vi "Main.vi"(0 "ON/OFF":bool, 1 "Slave Address":u8 max=127 step=1 format="%x", 2 "Data":u8[](array[numeric]) format="%x", 5 "Write":bool, 7 "Mode":T2, 9 "Addressing Mode":T1, 11 "Error in":errorcluster) -> (15 "Error out":errorcluster)   [LabVIEW 2020, in "I2C Module.lvlib"]
doc: "This is the main application of the I2C module library which is used to generate and acquire the data of the SDA and SCL lines which act as a bus"
uses:
  I2C Module.lvlib
  Typedefs/Modes of i2c.ctl
  Typedefs/Addressing modes.ctl
  Typedefs/Queue operations.ctl
  Typedefs/Data Cluster.ctl
  Typedefs/Cluster mode.ctl
  Typedefs/Cluster addressing.ctl
panel:
  out "Digital Waveform Graph":digitaldata(graph) caption="I2C DATA"
  in  "Voltage":dbl=1.8 min=1.8 max=5.0 step=0.1
  in  "Frequency":u32=10 min=10 max=100 step=1
  in  "Read":bool
  # "INTER-INTEGRATED-CIRCUIT MODULE"
  # "I2C a two wire interface for wired communication between devices where mostly single master and multiple slaves \nare connected for transmission and reception of data. Basically not more than 50 devices are connected as there \nwill be introduction of bus capacitance and further data loss."
  # "OFF"
  # "ON"
  # "KHz"
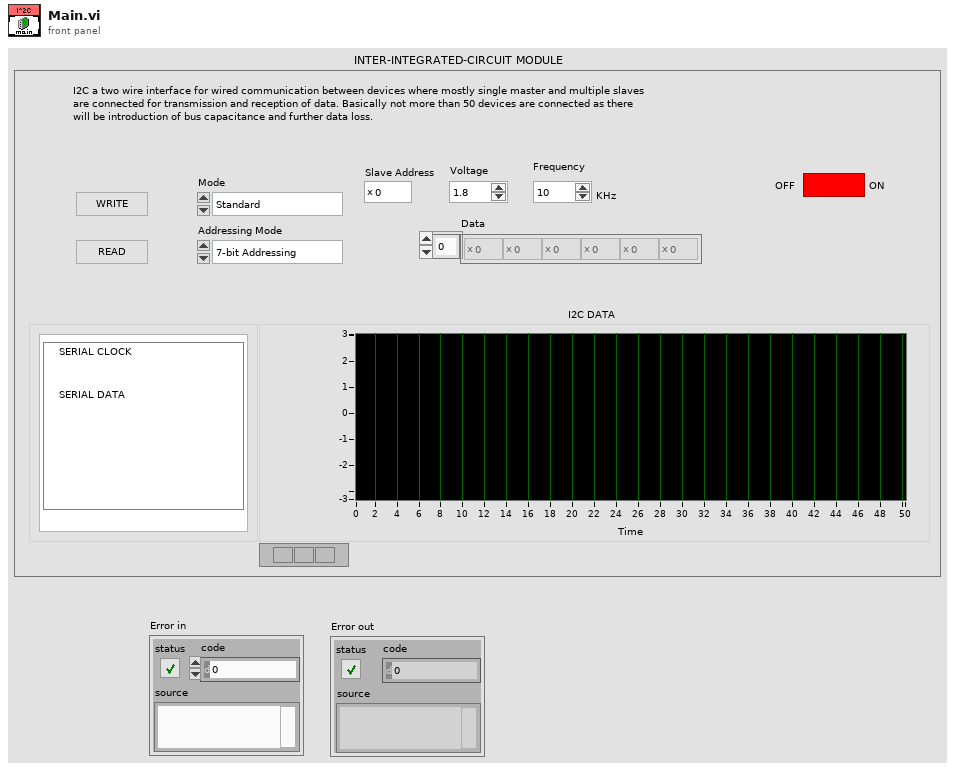
[diagram p1: front panel]
types:
  T1 = typedef "Addressing modes.ctl" = enum16{"7-bit Addressing", "10-bit Addressing"}
  T2 = typedef "Modes of i2c.ctl" = enum16{"Standard", "Fast Mode", "Fast Mode Plus"}
  T3 = typedef "Data Cluster.ctl" = cluster{"ON/OFF":bool, "Read":bool, "Stop":bool, "Ack":bool, "Nack":bool, "Mode":T4, "Addressing Mode":T5, "Frequency":u32, "Voltage":dbl, "SDA":bool[], "SCL":bool[], "Address":u8, "I2C DATA":dbl[], "I2C_DATA":dbl[][], "Enable":refnum<vi>[], "Disable":refnum<vi>[], "Write":bool, "I2C Digital":digitaldata, "Data":u8[], "Array update index":dbl}
  T4 = typedef "Cluster mode.ctl" = enum16{"Standard", "Fast Mode", "Fast Mode Plus"}
  T5 = typedef "Cluster addressing.ctl" = enum16{"7-bit Addressing", "10-bit Addressing"}
  T6 = typedef "I2C Module.lvlib/Queue operations.ctl" = enum16{"Create queue", " Enqueue N", "Enstack N", "Dequeue", "Flush", "Release"}
  T7 = enum8{"Enabled", "Disabled", "Disabled and Grayed Out"}
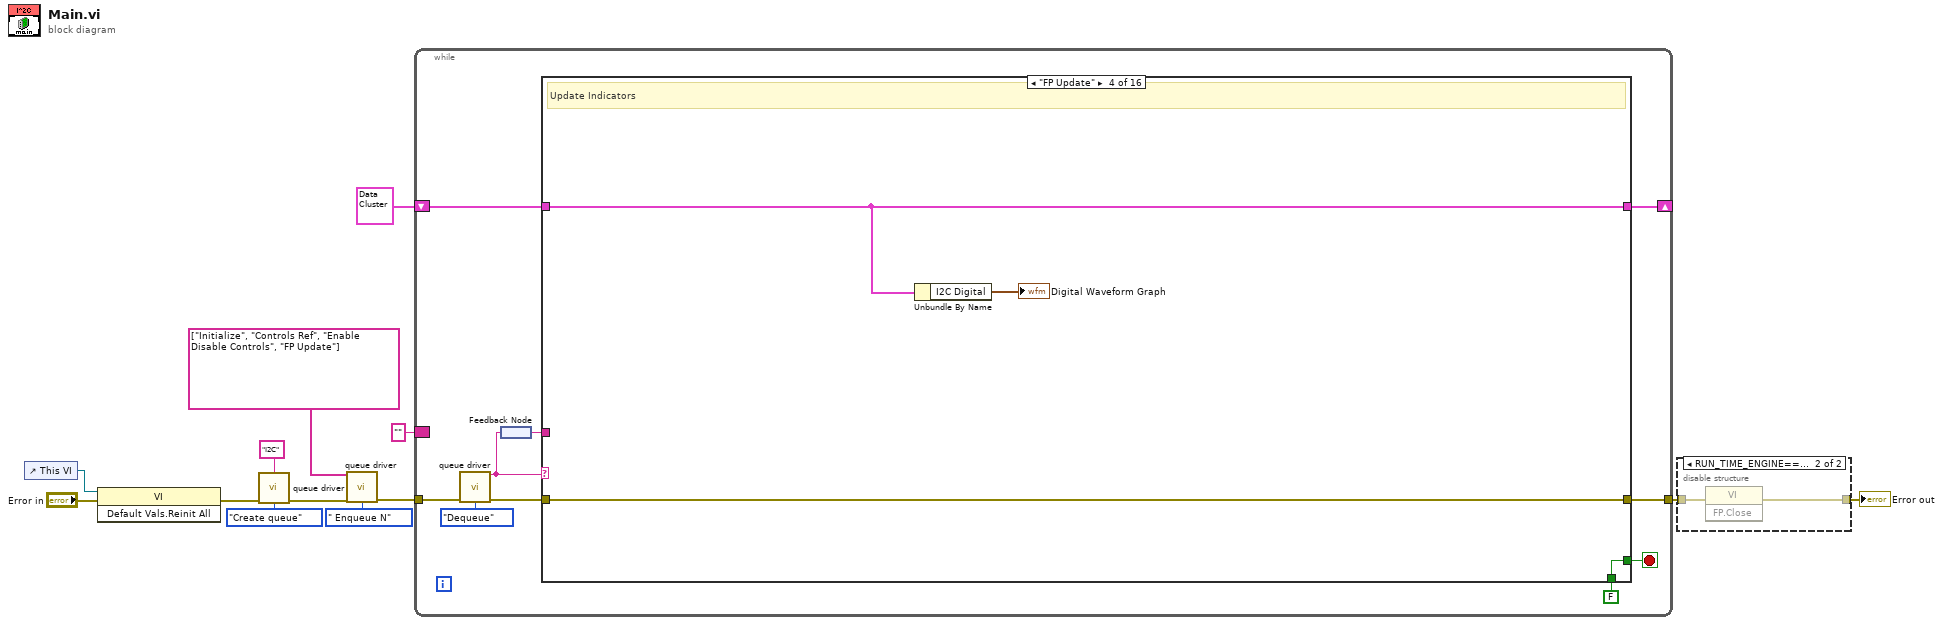
[diagram p0: block diagram]
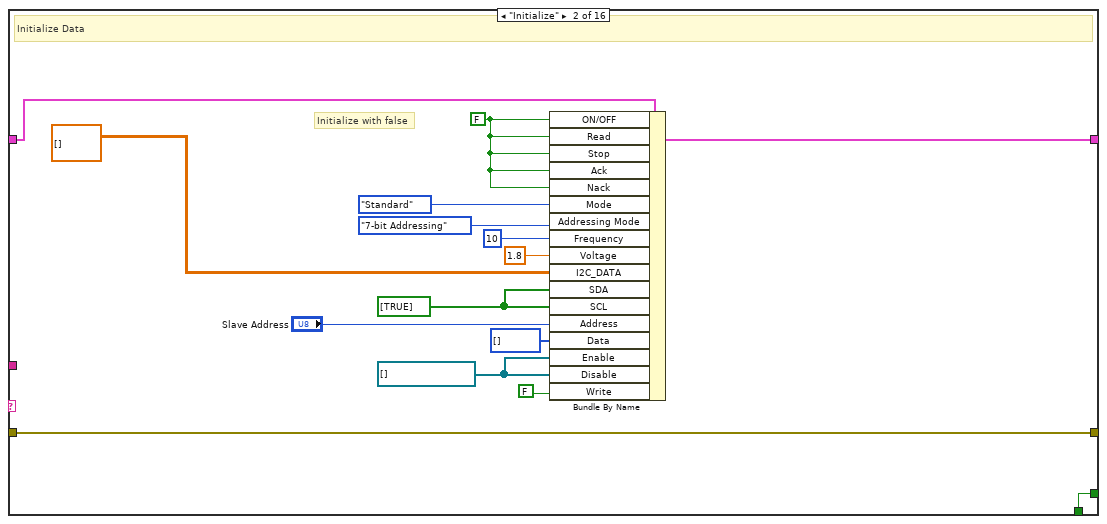
[diagram p4: hidden frame]
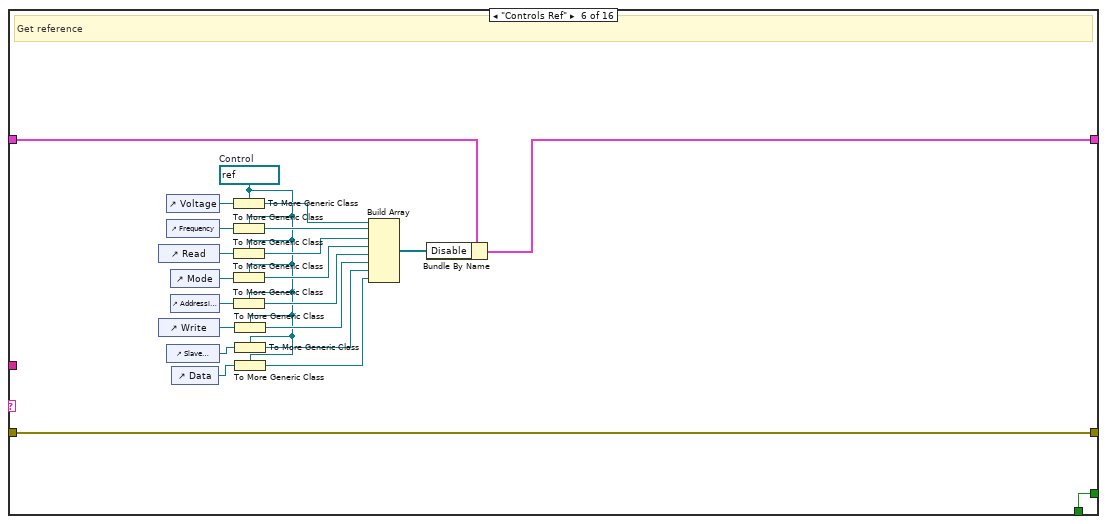
[diagram p7: hidden frame]
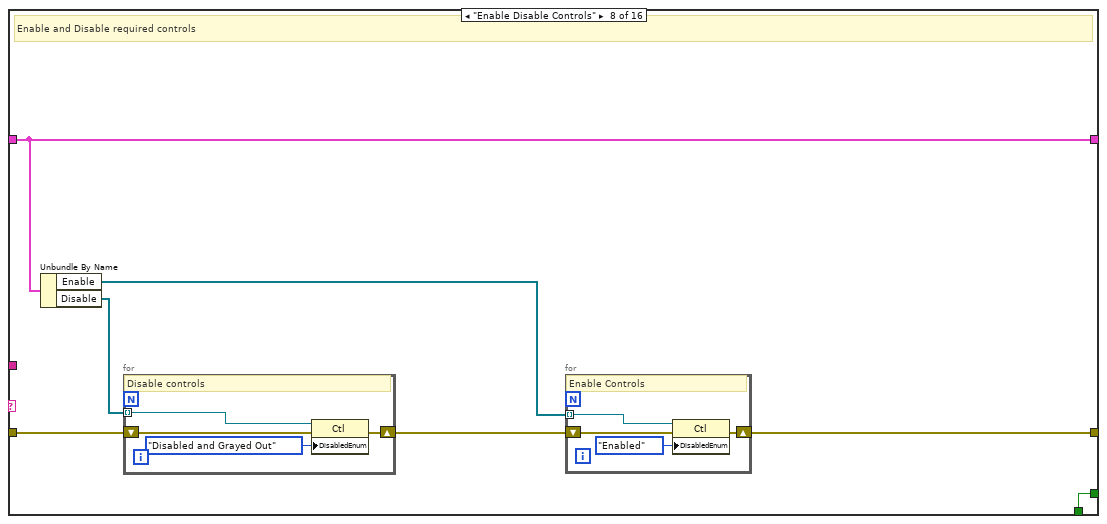
[diagram p9: hidden frame]
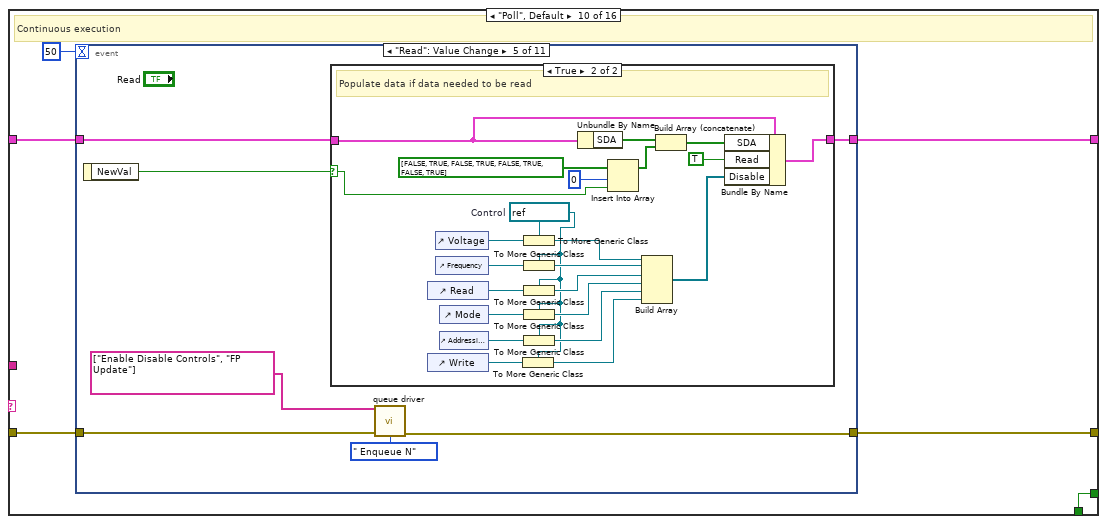
[diagram p11: hidden frame]
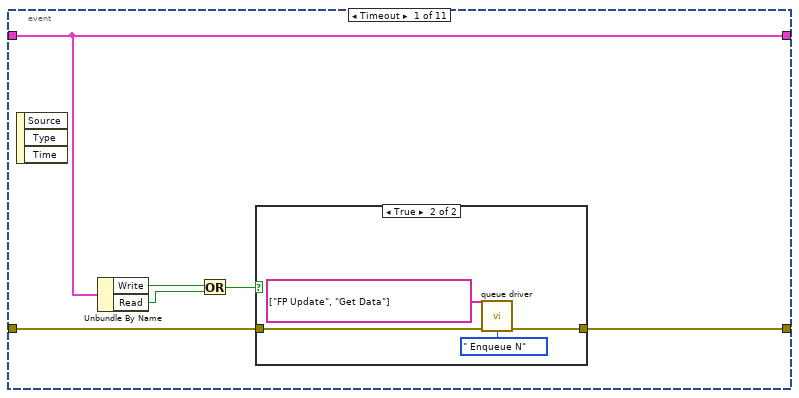
[diagram p12: hidden frame]
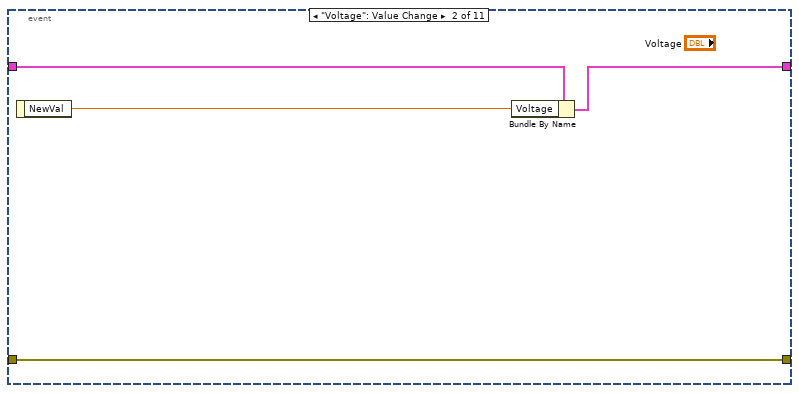
[diagram p14: hidden frame]
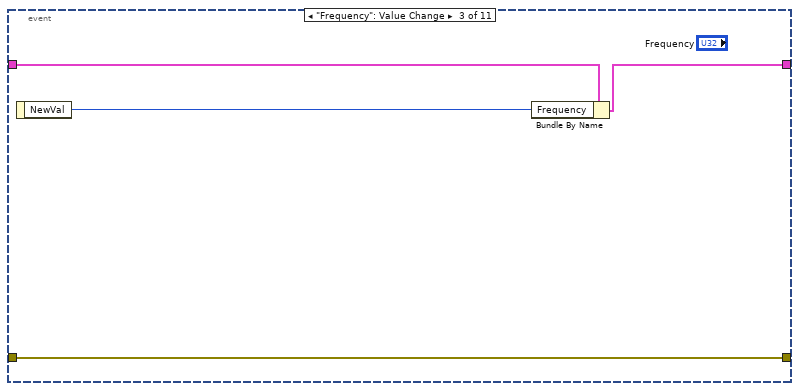
[diagram p15: hidden frame]
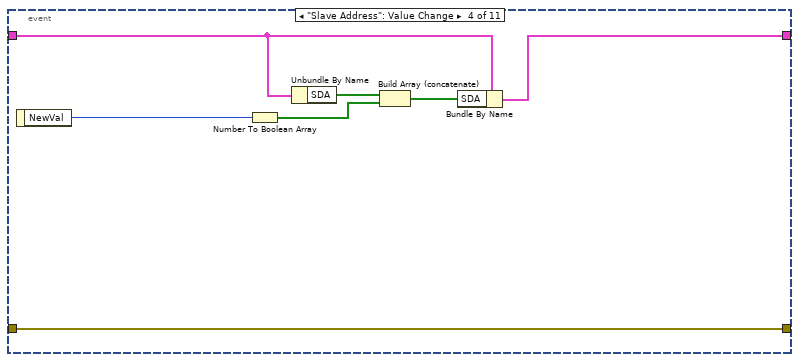
[diagram p16: hidden frame]
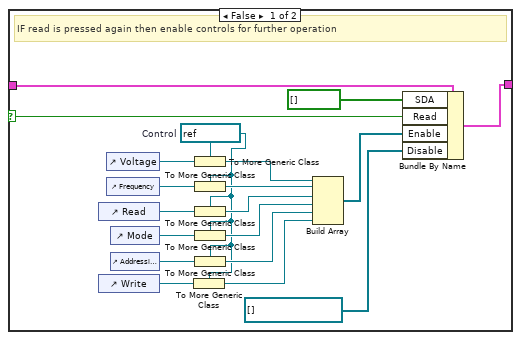
[diagram p17: hidden frame]
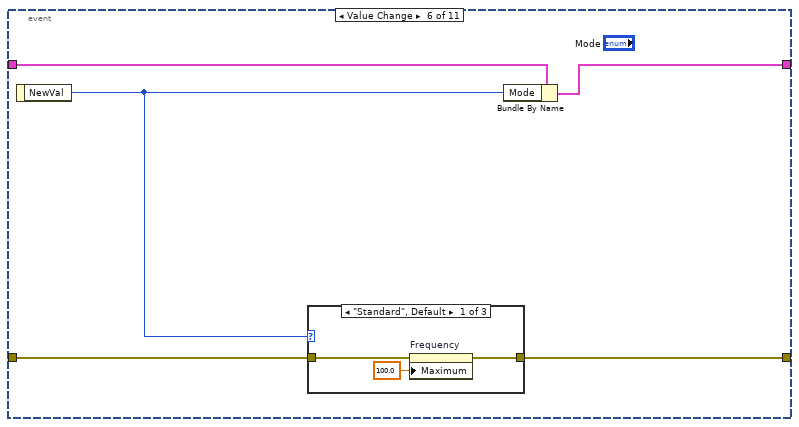
[diagram p18: hidden frame]
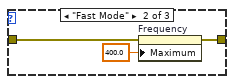
[diagram p19: hidden frame]
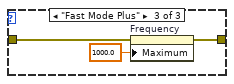
[diagram p20: hidden frame]
diagram:
  n1 = control-ref of="This VI"() -> (w12:refnum<vi>)
  n2 = invoke class="VI" method="Default Vals.Reinit All"(reference=w12, error in="Error in") -> (error out=w11:errorcluster)  [unwired: 1 in, 2 out]
  n3 = call "queue driver.vi"("Name"="I2C", "Error in"=w11, "Queue operations"=Queue_operations."Create queue") -> ("Error out"=w8:errorcluster)  [unwired: 11 in, 1 out]
  n4 = call "queue driver.vi"("Enqueue"=string[] ["Initialize", "Controls Ref", "Enable Disable Controls", "FP Update"], "Error in"=w8, "Queue operations"=Queue_operations." Enqueue N") -> ("Error out"=w6:errorcluster)  [unwired: 11 in, 1 out]
  n5 = while {
    tunnel: w6 -> [w22]
    border: "" ("Dequeued element") -> [_]
    tunnel: [w18] -> w2
    shift-right: [w15] -> _
    shift-left: T3 {"ON/OFF"=FALSE, "Read"=FALSE, "Stop"=FALSE, "Ack"=FALSE, "Nack"=FALSE, "Mode"=enum."Standard", "Addressing Mode"=enum."10-bit Addressing", "Frequency"=0, "Voltage"=0.0, "SDA"=[], "SCL"=[], "Address"=0, "I2C DATA"=[], "I2C_DATA"=[], "Enable"=[], "Disable"=[], "Write"=FALSE, "I2C Digital"={"transitions"=[], "data"=[]}, "Data"=[], "Array update index"=0.0} -> [w14]
    stop <- w17 stop-if-true
    n6 = call "queue driver.vi"("Error in"=w22, "Queue operations"=Queue_operations."Dequeue") -> ("Dequeued element"=w20:string, "Error out"=w19:errorcluster)  [unwired: 12 in]
    n7 = feedback-in #1(w20) -> ()
    n8 = feedback #1() -> (w21:string)
    n9 = case shown="\"FP Update\"" w20 {
      tunnel: w21 -> [_ _ _ _ _ _ _ _ _ _ _ _ _ w354 _ _]
      tunnel: w19 -> [w26 w41 w44 w48 w51 w73 w76 w81 w94 w98 w318 w341 w352 w356 w374 w379]
      tunnel: [w26 w41 w44 w48 w51 w73 w76 w80 w94 w99 w318 w341 w352 w355 w374 w377] -> w18
      tunnel: [w25 w40 w43 w47 w50 w72 w75 w83 w93 w97 w317 w340 w351 w366 w373 TRUE] -> w17
      tunnel: FALSE -> [w25 w40 w43 w47 w50 w72 w75 w83 w93 w97 w317 w340 w351 w366 w373 _]
      tunnel: [w24 w38 w42 w46 w49 w61 w74 w79 w92 w96 w316 w336 w350 w353 w372 w375] -> w15
      tunnel: w14 -> [w24 w39 w42 w46 w49 w62 w74 w79 w92 w95 w316 w337 w350 w353 w372 w375]
      frame "/***Initialize***/" {
      }
      frame "Initialize" {
        w28 = refnum<vi>[] [] ("Enable")
        w29 = bool[] [TRUE] ("SCL")
        w37 = FALSE ("ON/OFF")
        # "Initialize with false"
        # "Initialize Data"
        n10 = Bundle By Name(cluster=w39, "ON/OFF"=w37, "Read"=w37, "Stop"=w37, "Ack"=w37, "Nack"=w37, "Mode"=Cluster_mode."Standard", "Addressing Mode"=Cluster_addressing."7-bit Addressing", "Frequency"=u32 10, "Voltage"=1.8, "I2C_DATA"=dbl[][] [] ("x*y"), "SDA"=w29, "SCL"=w29, "Address"="Slave Address", "Data"=u8[] [], "Enable"=w28, "Disable"=w28, "Write"=FALSE ("Read/ Write")) -> (w38:T3)
      }
      frame "/***FP Related***/" {
      }
      frame "FP Update" {
        # "Update Indicators"
        n11 = Unbundle By Name(w46) -> ("I2C Digital"=→"Digital Waveform Graph":digitaldata)
      }
      frame "/***Controls ref***/" {
      }
      frame "Controls Ref" {
        w54 = refnum<vi> refnum  # Control
        # "Get reference"
        n12 = control-ref of="Read"() -> (w69:refnum<vi>)
        n13 = control-ref of="Write"() -> (w58:refnum<vi>)
        n14 = control-ref of="Voltage"() -> (w71:refnum<vi>)
        n15 = control-ref of="Frequency"() -> (w70:refnum<vi>)
        n16 = control-ref of="Slave Address"() -> (w56:refnum<vi>)
        n17 = control-ref of="Mode"() -> (w68:refnum<vi>)
        n18 = control-ref of="Addressing Mode"() -> (w67:refnum<vi>)
        n19 = control-ref of="Data"() -> (w55:refnum<vi>)
        n20 = To More Generic Class(target class=w54, reference=w71) -> (generic class reference=w66:refnum<vi>)
        n21 = To More Generic Class(target class=w54, reference=w70) -> (generic class reference=w65:refnum<vi>)
        n22 = To More Generic Class(target class=w54, reference=w69) -> (generic class reference=w64:refnum<vi>)
        n23 = To More Generic Class(target class=w54, reference=w68) -> (generic class reference=w63:refnum<vi>)
        n24 = To More Generic Class(target class=w54, reference=w67) -> (generic class reference=w59:refnum<vi>)
        n25 = To More Generic Class(target class=w54, reference=w58) -> (generic class reference=w57:refnum<vi>)
        n26 = To More Generic Class(target class=w54, reference=w56) -> (generic class reference=w53:refnum<vi>)
        n27 = To More Generic Class(target class=w54, reference=w55) -> (generic class reference=w52:refnum<vi>)
        n28 = Build Array(w66, w65, w64, w63, w59, w57, w53, w52) -> (w60:refnum<vi>[])
        n29 = Bundle By Name(cluster=w62, "Disable"=w60) -> (w61:T3)
      }
      frame "/***Enable Disable Controls***/" {
      }
      frame "Enable Disable Controls" {
        # "Enable and Disable required controls"
        n30 = Unbundle By Name(w79) -> ("Enable"=w78:refnum<vi>[], "Disable"=w77:refnum<vi>[])
        n31 = for {
          shift-right: [w90] -> w82
          shift-left: w81 -> [w91]
          tunnel: w77 -> [w88] mode=indexing
          # "Disable controls"
          n32 = property class="Ctl"(reference=w88, error in=w91, "DisabledEnum"=T7."Disabled and Grayed Out" ("Disabled")) -> (error out=w90:errorcluster)  [unwired: 1 out]
        }
        n33 = for {
          shift-right: [w86] -> w80
          shift-left: w82 -> [w87]
          tunnel: w78 -> [w84] mode=indexing
          # "Enable Controls"
          n34 = property class="Ctl"(reference=w84, error in=w87, "DisabledEnum"=T7."Enabled" ("Disabled")) -> (error out=w86:errorcluster)  [unwired: 1 out]
        }
      }
      frame "/***Application***/" {
      }
      frame "Poll", Default {
        # "Continuous execution"
        n35 = event shown="[4] \"Read\": Value Change" {
          selector: _ -> [_ _ _ _ _ _ _ _ _ _ _]
          dyn-events: _ -> [_ _ _ _ _ _ _ _ _ _ _]
          timeout: 50 -> [_ _ _ _ _ _ _ _ _ _ _]
          tunnel: [w105 w115 w119 w126 w128 w176 w193 w197 w241 w245 w311] -> w99
          tunnel: w98 -> [w106 w115 w119 w126 w129 w177 w193 w198 w241 w246 w312]
          tunnel: [w104 w113 w117 w123 w133 w179 w191 w200 w239 w242 w295] -> w96
          tunnel: w95 -> [w104 w114 w118 w124 w132 w180 w192 w194 w240 w243 w296]
          event Timeout {
            n36 = event-data() -> ()  [unwired: 1 in, 3 out]
            n37 = Unbundle By Name(w104) -> ("Write"=w103:bool, "Read"=w102:bool)
            n38 = Or(x=w103, y=w102) -> (x .or. y?=w101:bool)
            n39 = case shown="True" w101 {
              tunnel: w106 -> [w107 w110]
              tunnel: [w107 w109] -> w105
              frame False {
              }
              frame True {
                n40 = call "queue driver.vi"("Enqueue"=string[] ["FP Update", "Get Data"], "Error in"=w110, "Queue operations"=Queue_operations." Enqueue N") -> ("Error out"=w109:errorcluster)  [unwired: 11 in, 1 out]
              }
            }
          }
          event "Voltage": Value Change {
            n41 = event-data() -> ("NewVal"=w112:dbl)  [unwired: 1 in]
            n42 = Bundle By Name(cluster=w114, "Voltage"=w112) -> (w113:T3)
          }
          event "Frequency": Value Change {
            n43 = event-data() -> ("NewVal"=w116:u32)  [unwired: 1 in]
            n44 = Bundle By Name(cluster=w118, "Frequency"=w116) -> (w117:T3)
          }
          event "Slave Address": Value Change {
            n45 = event-data() -> ("NewVal"=w125:u8)  [unwired: 1 in]
            n46 = Number To Boolean Array(number=w125) -> (Boolean array=w120:bool[])
            n47 = Unbundle By Name(w124) -> ("SDA"=w122:bool[])
            n48 = Build Array (concatenate)(w122, w120) -> (w121:bool[])
            n49 = Bundle By Name(cluster=w124, "SDA"=w121) -> (w123:T3)
          }
          event "Read": Value Change {
            n50 = event-data() -> ("NewVal"=w131:bool)  [unwired: 1 in]
            n51 = case shown="True" w131 {
              selector: w131 -> [w150 w167]
              tunnel: [w151 w175] -> w133
              tunnel: w132 -> [w152 w168]
              frame False {
                w136 = refnum<vi> refnum  # Control
                # "IF read is pressed again then enable controls for further operation"
                n52 = control-ref of="Read"() -> (w139:refnum<vi>)
                n53 = control-ref of="Write"() -> (w147:refnum<vi>)
                n54 = control-ref of="Voltage"() -> (w141:refnum<vi>)
                n55 = control-ref of="Frequency"() -> (w140:refnum<vi>)
                n56 = control-ref of="Mode"() -> (w138:refnum<vi>)
                n57 = control-ref of="Addressing Mode"() -> (w137:refnum<vi>)
                n58 = To More Generic Class(target class=w136, reference=w147) -> (generic class reference=w148:refnum<vi>)
                n59 = To More Generic Class(target class=w136, reference=w141) -> (generic class reference=w146:refnum<vi>)
                n60 = To More Generic Class(target class=w136, reference=w140) -> (generic class reference=w145:refnum<vi>)
                n61 = To More Generic Class(target class=w136, reference=w139) -> (generic class reference=w144:refnum<vi>)
                n62 = To More Generic Class(target class=w136, reference=w138) -> (generic class reference=w143:refnum<vi>)
                n63 = To More Generic Class(target class=w136, reference=w137) -> (generic class reference=w142:refnum<vi>)
                n64 = Build Array(w146, w145, w144, w143, w142, w148) -> (w135:refnum<vi>[])
                n65 = Bundle By Name(cluster=w152, "SDA"=bool[] [], "Read"=w150, "Enable"=w135, "Disable"=refnum<vi>[] []) -> (w151:T3)
              }
              frame True {
                w154 = refnum<vi> refnum  # Control
                # "Populate data if data needed to be read"
                n66 = control-ref of="Read"() -> (w157:refnum<vi>)
                n67 = control-ref of="Write"() -> (w165:refnum<vi>)
                n68 = control-ref of="Voltage"() -> (w159:refnum<vi>)
                n69 = control-ref of="Frequency"() -> (w158:refnum<vi>)
                n70 = control-ref of="Mode"() -> (w156:refnum<vi>)
                n71 = control-ref of="Addressing Mode"() -> (w155:refnum<vi>)
                n72 = To More Generic Class(target class=w154, reference=w165) -> (generic class reference=w166:refnum<vi>)
                n73 = To More Generic Class(target class=w154, reference=w159) -> (generic class reference=w164:refnum<vi>)
                n74 = To More Generic Class(target class=w154, reference=w158) -> (generic class reference=w163:refnum<vi>)
                n75 = To More Generic Class(target class=w154, reference=w157) -> (generic class reference=w162:refnum<vi>)
                n76 = To More Generic Class(target class=w154, reference=w156) -> (generic class reference=w161:refnum<vi>)
                n77 = To More Generic Class(target class=w154, reference=w155) -> (generic class reference=w160:refnum<vi>)
                n78 = Unbundle By Name(w168) -> ("SDA"=w174:bool[])
                n79 = Insert Into Array(array=bool[] [FALSE, TRUE, FALSE, TRUE, FALSE, TRUE, FALSE, TRUE] ("SDA"), index=0, new element=w167) -> (w170:bool[])
                n80 = Build Array(w164, w163, w162, w161, w160, w166) -> (w153:refnum<vi>[])
                n81 = Build Array (concatenate)(w174, w170) -> (w173:bool[])
                n82 = Bundle By Name(cluster=w168, "SDA"=w173, "Read"=TRUE ("Read/ Write"), "Disable"=w153) -> (w175:T3)
              }
            }
            n83 = call "queue driver.vi"("Enqueue"=string[] ["Enable Disable Controls", "FP Update"], "Error in"=w129, "Queue operations"=Queue_operations." Enqueue N") -> ("Error out"=w128:errorcluster)  [unwired: 11 in, 1 out]
          }
          event Value Change {
            n84 = event-data() -> ("NewVal"=w178:T2)  [unwired: 1 in]
            n85 = case shown="\"Standard\", Default" w178 {
              tunnel: w177 -> [w183 w186 w189]
              tunnel: [w182 w185 w188] -> w176
              frame "Standard", Default {
                n86 = property on="Frequency" class="DigNum (strict)"(error in=w183, "Maximum"=100.0 ("Data Entry Limits:Maximum")) -> (error out=w182:errorcluster)  [unwired: 1 in, 1 out]
              }
              frame "Fast Mode" {
                n87 = property on="Frequency" class="DigNum (strict)"(error in=w186, "Maximum"=400.0 ("Data Entry Limits:Maximum")) -> (error out=w185:errorcluster)  [unwired: 1 in, 1 out]
              }
              frame "Fast Mode Plus" {
                n88 = property on="Frequency" class="DigNum (strict)"(error in=w189, "Maximum"=1000.0 ("Data Entry Limits:Maximum")) -> (error out=w188:errorcluster)  [unwired: 1 in, 1 out]
              }
            }
            n89 = Bundle By Name(cluster=w180, "Mode"=w178) -> (w179:T3)
          }
          event Value Change {
            n90 = event-data() -> ("NewVal"=w190:T1)  [unwired: 1 in]
            n91 = Bundle By Name(cluster=w192, "Addressing Mode"=w190) -> (w191:T3)
          }
          event "Write": Value Change {
            n92 = event-data() -> ("NewVal"=w195:bool)  [unwired: 1 in]
            n93 = case shown="True" w195 {
              selector: w195 -> [w205 w222]
              tunnel: [w212 w236] -> w200
              tunnel: w194 -> [w206 w221]
              frame False {
                w203 = refnum<vi> refnum  # Control
                n94 = control-ref of="Read"() -> (w209:refnum<vi>)
                n95 = control-ref of="Write"() -> (w204:refnum<vi>)
                n96 = control-ref of="Voltage"() -> (w211:refnum<vi>)
                n97 = control-ref of="Frequency"() -> (w210:refnum<vi>)
                n98 = control-ref of="Mode"() -> (w208:refnum<vi>)
                n99 = control-ref of="Addressing Mode"() -> (w207:refnum<vi>)
                n100 = To More Generic Class(target class=w203, reference=w204) -> (generic class reference=w202:refnum<vi>)
                n101 = To More Generic Class(target class=w203, reference=w211) -> (generic class reference=w218:refnum<vi>)
                n102 = To More Generic Class(target class=w203, reference=w210) -> (generic class reference=w217:refnum<vi>)
                n103 = To More Generic Class(target class=w203, reference=w209) -> (generic class reference=w216:refnum<vi>)
                n104 = To More Generic Class(target class=w203, reference=w208) -> (generic class reference=w215:refnum<vi>)
                n105 = To More Generic Class(target class=w203, reference=w207) -> (generic class reference=w214:refnum<vi>)
                n106 = Build Array(w218, w217, w216, w215, w214, w202) -> (w219:refnum<vi>[])
                n107 = Bundle By Name(cluster=w206, "Write"=w205, "Enable"=w219, "Disable"=refnum<vi>[] [], "Data"=u8[] []) -> (w212:T3)
              }
              frame True {
                w230 = refnum<vi> refnum  # Control
                n108 = Unbundle By Name(w221) -> ("Data"=w220:u8[])
                n109 = control-ref of="Read"() -> (w227:refnum<vi>)
                n110 = control-ref of="Voltage"() -> (w229:refnum<vi>)
                n111 = control-ref of="Frequency"() -> (w228:refnum<vi>)
                n112 = control-ref of="Mode"() -> (w226:refnum<vi>)
                n113 = control-ref of="Addressing Mode"() -> (w225:refnum<vi>)
                n114 = To More Generic Class(target class=w230, reference=w229) -> (generic class reference=w231:refnum<vi>)
                n115 = To More Generic Class(target class=w230, reference=w228) -> (generic class reference=w232:refnum<vi>)
                n116 = To More Generic Class(target class=w230, reference=w227) -> (generic class reference=w233:refnum<vi>)
                n117 = To More Generic Class(target class=w230, reference=w226) -> (generic class reference=w234:refnum<vi>)
                n118 = To More Generic Class(target class=w230, reference=w225) -> (generic class reference=w235:refnum<vi>)
                n119 = Build Array(w231, w232, w233, w234, w235) -> (w224:refnum<vi>[])
                n120 = Bundle By Name(cluster=w221, "Write"=w222, "Disable"=w224, "Enable"=refnum<vi>[] [] ("Disable"), "Data"=w220) -> (w236:T3)
              }
            }
            n121 = call "queue driver.vi"("Enqueue"=string[] ["Enable Disable Controls", "FP Update"], "Error in"=w198, "Queue operations"=Queue_operations." Enqueue N") -> ("Error out"=w197:errorcluster)  [unwired: 11 in, 1 out]
          }
          event "Data": Value Change {
            n122 = event-data() -> ("NewVal"=w238:u8[])  [unwired: 1 in]
            n123 = Bundle By Name(cluster=w240, "Data"=w238, "Array update index"=0.0) -> (w239:T3)
          }
          event "ON/OFF": Value Change {
            n124 = event-data() -> ("NewVal"=w244:bool)  [unwired: 1 in]
            n125 = case shown="False" w244 {
              tunnel: w246 -> [w269 w279]
              tunnel: [w268 w278] -> w245
              tunnel: w243 -> [w253 w284]
              tunnel: [w254 w282] -> w242
              frame False {
                w249 = refnum<vi> refnum  # Control
                n126 = control-ref of="Read"() -> (w258:refnum<vi>)
                n127 = control-ref of="Write"() -> (w255:refnum<vi>)
                n128 = control-ref of="Slave Address"() -> (w251:refnum<vi>)
                n129 = control-ref of="Data"() -> (w250:refnum<vi>)
                n130 = control-ref of="Voltage"() -> (w260:refnum<vi>)
                n131 = control-ref of="Frequency"() -> (w259:refnum<vi>)
                n132 = control-ref of="Mode"() -> (w257:refnum<vi>)
                n133 = control-ref of="Addressing Mode"() -> (w256:refnum<vi>)
                n134 = To More Generic Class(target class=w249, reference=w251) -> (generic class reference=w248:refnum<vi>)
                n135 = To More Generic Class(target class=w249, reference=w250) -> (generic class reference=w247:refnum<vi>)
                n136 = To More Generic Class(target class=w249, reference=w260) -> (generic class reference=w266:refnum<vi>)
                n137 = To More Generic Class(target class=w249, reference=w259) -> (generic class reference=w265:refnum<vi>)
                n138 = To More Generic Class(target class=w249, reference=w258) -> (generic class reference=w264:refnum<vi>)
                n139 = To More Generic Class(target class=w249, reference=w257) -> (generic class reference=w263:refnum<vi>)
                n140 = To More Generic Class(target class=w249, reference=w256) -> (generic class reference=w262:refnum<vi>)
                n141 = To More Generic Class(target class=w249, reference=w255) -> (generic class reference=w261:refnum<vi>)
                n142 = Build Array(w266, w265, w264, w263, w262, w261, w248, w247) -> (w252:refnum<vi>[])
                n143 = call "queue driver.vi"("Enqueue"=string[] ["Enable Disable Controls", "Exit"], "Error in"=w269, "Queue operations"=Queue_operations." Enqueue N") -> ("Error out"=w268:errorcluster)  [unwired: 11 in, 1 out]
                n144 = Bundle By Name(cluster=w253, "Enable"=w252) -> (w254:T3)
              }
              frame True {
                w275 = refnum<vi> refnum  # Control
                n145 = control-ref of="Read"() -> (w287:refnum<vi>)
                n146 = control-ref of="Write"() -> (w277:refnum<vi>)
                n147 = control-ref of="Voltage"() -> (w289:refnum<vi>)
                n148 = control-ref of="Frequency"() -> (w288:refnum<vi>)
                n149 = control-ref of="Slave Address"() -> (w274:refnum<vi>)
                n150 = control-ref of="Mode"() -> (w286:refnum<vi>)
                n151 = control-ref of="Addressing Mode"() -> (w285:refnum<vi>)
                n152 = control-ref of="Data"() -> (w273:refnum<vi>)
                n153 = To More Generic Class(target class=w275, reference=w289) -> (generic class reference=w294:refnum<vi>)
                n154 = To More Generic Class(target class=w275, reference=w288) -> (generic class reference=w293:refnum<vi>)
                n155 = To More Generic Class(target class=w275, reference=w287) -> (generic class reference=w292:refnum<vi>)
                n156 = To More Generic Class(target class=w275, reference=w286) -> (generic class reference=w291:refnum<vi>)
                n157 = To More Generic Class(target class=w275, reference=w285) -> (generic class reference=w290:refnum<vi>)
                n158 = To More Generic Class(target class=w275, reference=w277) -> (generic class reference=w276:refnum<vi>)
                n159 = To More Generic Class(target class=w275, reference=w274) -> (generic class reference=w272:refnum<vi>)
                n160 = To More Generic Class(target class=w275, reference=w273) -> (generic class reference=w271:refnum<vi>)
                n161 = call "queue driver.vi"("Enqueue"=string[] ["Enable Disable Controls"], "Error in"=w279, "Queue operations"=Queue_operations." Enqueue N") -> ("Error out"=w278:errorcluster)  [unwired: 11 in, 1 out]
                n162 = Build Array(w294, w293, w292, w291, w290, w276, w272, w271) -> (w283:refnum<vi>[])
                n163 = Bundle By Name(cluster=w284, "Enable"=w283) -> (w282:T3)
              }
            }
          }
          event Panel Close? {
            w297 = refnum<vi> refnum  # Control
            n164 = event-data() -> ()  [unwired: 1 in, 1 out]
            n165 = control-ref of="Read"() -> (w302:refnum<vi>)
            n166 = control-ref of="Write"() -> (w299:refnum<vi>)
            n167 = control-ref of="Voltage"() -> (w304:refnum<vi>)
            n168 = control-ref of="Frequency"() -> (w303:refnum<vi>)
            n169 = control-ref of="Mode"() -> (w301:refnum<vi>)
            n170 = control-ref of="Addressing Mode"() -> (w300:refnum<vi>)
            n171 = To More Generic Class(target class=w297, reference=w304) -> (generic class reference=w310:refnum<vi>)
            n172 = To More Generic Class(target class=w297, reference=w303) -> (generic class reference=w309:refnum<vi>)
            n173 = To More Generic Class(target class=w297, reference=w302) -> (generic class reference=w308:refnum<vi>)
            n174 = To More Generic Class(target class=w297, reference=w301) -> (generic class reference=w307:refnum<vi>)
            n175 = To More Generic Class(target class=w297, reference=w300) -> (generic class reference=w306:refnum<vi>)
            n176 = To More Generic Class(target class=w297, reference=w299) -> (generic class reference=w305:refnum<vi>)
            n177 = call "queue driver.vi"("Enqueue"=string[] ["Enable Disable Controls", "Exit"], "Error in"=w312, "Queue operations"=Queue_operations." Enqueue N") -> ("Error out"=w311:errorcluster)  [unwired: 11 in, 1 out]
            n178 = Build Array(w310, w309, w308, w307, w306, w305) -> (w298:refnum<vi>[])
            n179 = Bundle By Name(cluster=w296, "Enable"=w298) -> (w295:T3)
            n180 = event-data("Discard?"=TRUE) -> ()  [unwired: 1 in, 1 out]
          }
        }
      }
      frame "/***Get Data***/" {
      }
      frame "Get Data" {
        # "Transmit and Receive Bus Data"
        n181 = Unbundle By Name(w337) -> ("Voltage"=w338:dbl, "SDA"=w339:bool[], "Data"=w328:u8[], "SCL"=w334:bool[], "Array update index"=w329:dbl)
        n182 = Array Size(array=w328) -> (size(s)=w327:i32)
        n183 = To Double Precision Float(number=w327) -> (double precision float=w326:dbl)
        n184 = Less Or Equal?(x=w329, y=w326) -> (x <= y?=w319:bool)
        n185 = case shown="True" w319 {
          tunnel: w339 -> [w342 w349]
          tunnel: [w342 w348] -> w332
          tunnel: w328 -> [_ w347]
          frame False {
          }
          frame True {
            n186 = Index Array(array=w347) -> (element=w346:u8)  [unwired: 1 in]
            n187 = Number To Boolean Array(number=w346) -> (Boolean array=w345:bool[])
            n188 = Insert Into Array(array=w345, new element=FALSE ("new element/subarray")) -> (w343:bool[])  [unwired: 1 in]
            n189 = Build Array (concatenate)(w349, w343) -> (w348:bool[])
          }
        }
        n190 = Build Array (concatenate)(w334, bool[] [FALSE, TRUE, FALSE, TRUE, FALSE, TRUE, FALSE, TRUE] ("element")) -> (w333:bool[])
        n191 = Build Array(w332, w333) -> (w325:bool[][])
        n192 = Increment(x=w329) -> (x+1=w330:dbl)
        n193 = Boolean To (0,1)(Boolean=w325) -> (0, 1=w322:i16[][])
        n194 = To Double Precision Float(number=w322) -> (double precision float=w324:dbl[][])
        n195 = To Unsigned Byte Integer(number=w322) -> (unsigned 8bit integer=w321:u8[][])
        n196 = Transpose 2D Array(2D array=w321) -> (transposed array=w320:u8[][])
        n197 = Multiply(x=w338, y=w324) -> (x*y=w335:dbl[][])
        n198 = Bundle By Name("data"=w320) -> (w331:digitaldata)  [unwired: 1 in]
        n199 = Bundle By Name(cluster=w337, "SDA"=w332, "I2C_DATA"=w335, "SCL"=w333, "I2C Digital"=w331, "Array update index"=w330) -> (w336:T3)
      }
      frame "/***Error***/" {
      }
      frame "Error" {
        # "Pop up if Error"
        n200 = Unbundle By Name(w356) -> ("code"=w363:i32, "source"=w362:string)
        n201 = call <vilib>:"Clear Errors.vi"("error in (no error)"=w356, "specific error code to clear (0: all)"=w363) -> ("error out"=w365:errorcluster)  [unwired: 4 in, 1 out]
        n202 = Format Into String(format string="Error occurred in state \"%s\"!!\nError Code: %d\nError Source: %s\n\nDo you wish to continue?", error in=w365, w354, w363, w362) -> (resulting string=w361:string, error out=w358:errorcluster)  [unwired: 1 in]
        n203 = Two Button Dialog(message=w361, 1:"Exit" ("F button name (\"Cancel\")"), 2:"Continue" ("T button name (\"OK\")")) -> (T button?=w357:bool)
        n204 = case shown="False" w357 {
          tunnel: w358 -> [w369 w371]
          tunnel: [w368 w371] -> w355
          frame False {
            # "Exit"
            n205 = call "queue driver.vi"("Enqueue"=string[] ["Exit"], "Error in"=w369, "Queue operations"=Queue_operations." Enqueue N") -> ("Error out"=w368:errorcluster)  [unwired: 11 in, 1 out]
          }
          frame True {
            # "Continue"
          }
        }
      }
      frame "/***Exit***/" {
      }
      frame "Exit" {
        # "Flush and Release Queue"
        # "Terminate execution"
        n206 = call "queue driver.vi"("Error in"=w379, "Queue operations"=Queue_operations."Flush") -> ("Error out"=w378:errorcluster)  [unwired: 12 in, 1 out]
        n207 = call "queue driver.vi"("Error in"=w378, "Queue operations"=Queue_operations."Release") -> ("Error out"=w377:errorcluster)  [unwired: 12 in, 1 out]
      }
    }
  }
  n208 = disable-structure shown="RUN_TIME_ENGINE==True" {
    disable-tunnel: w2 -> [w382 w384]
    disable-tunnel: [w382 w383] -> w1
    frame condition #0 (active) {
    }
    frame condition #1 {
      n209 = invoke class="VI" method="FP.Close"(error in=w384) -> (error out=w383:errorcluster)  [unwired: 2 in, 2 out]
    }
  }
  "Error out" <- w1
